vi "Stop Impl.vi"(11 "Thorlabs Power Meter in":refnum<class "Thorlabs Power Meter.lvclass">) -> (3 "Thorlabs Power Meter out":refnum<class "Thorlabs Power Meter.lvclass">)   [LabVIEW 2023, in "Thorlabs Power Meter.lvlib" / "Thorlabs Power Meter.lvclass"]
uses:
  Thorlabs Power Meter.lvclass
  Thorlabs Power Meter.lvclass/Thorlabs Power Meter.ctl
  Thorlabs Power Meter.lvlib
panel:
  out "error out":errorcluster
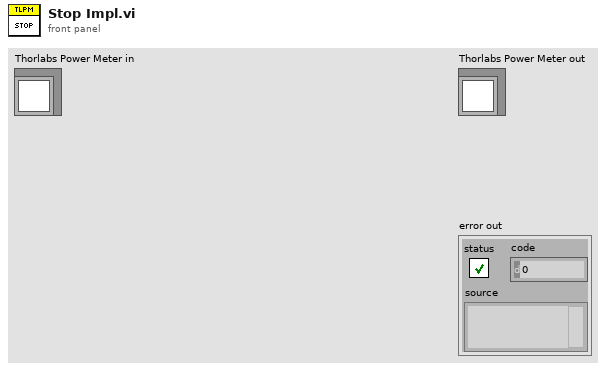
[diagram p1: front panel]
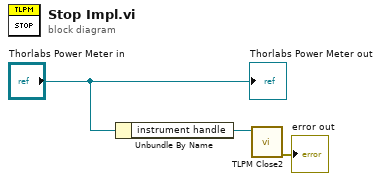
[diagram p0: block diagram]
diagram:
  n1 = Unbundle By Name("Thorlabs Power Meter in") -> ("instrument handle"=w2:refnum<visa-resource-name>)
  n2 = call "TLPM Close2.vi"("instrument handle"=w2) -> ("error out"=→"error out":errorcluster)  [unwired: 10 in]
  "Thorlabs Power Meter out" <- "Thorlabs Power Meter in"
